vi "Nominal LabVIEW Client API Tree.vi"() -> ()   [LabVIEW 2020]
doc: "This VI is intentionally non-runnable and is designed purely for reference and documentation purposes."
uses:
  Nominal Client.lvclass
  76682c19-609f-4d4f-aff0-eacf46784d00.vi
  2ed37eeb-a64f-4a91-b3eb-4b67bea1485f.vi
  95585ae7-5aba-4d79-b365-cf4aec99f37a.vi
  cba89ab2-b70c-4f15-9195-c2a6f1b0cacd.vi
  95564017-f1d2-4f01-914a-473868c7473e.vi
  f4306f34-5195-4845-a7f4-29a524f2fbc4.vi
  Nominal Client MultiPart Upload/Multipart Upload.lvclass
  timestampMetadata/timestampMetadata.lvclass
  78d8da57-746a-4171-a186-1f17ed8bf924.vi
  ts.epochOfTimeUnit/build.epoch.vi
  ts.epochOfTimeUnit/ts.epochOfTimeUnit.lvclass
  03991706-e7ff-4459-af3d-5364ac0de598.vi
  f1e9a693-645c-4611-911e-4c295cbd5176.vi
  catalog.wait_until_ingest_complete.vi
  ingest_csv.vi
  upload_ingest.csv.vi
  upload_ingest.video.vi
  stream_custom_cluster/stream_custom_cluster.lvclass
  type/type.lvclass
  asset/asset.lvclass
  Run/Run.lvclass
panel:
  in  "Title":string
  in  "data cluster":T1={"Value"=3.14159, "Nanoseconds"=0, "status"=""}
  in  "Description":string
  in  "Dataset Name":string
  # "See Block Diagram"
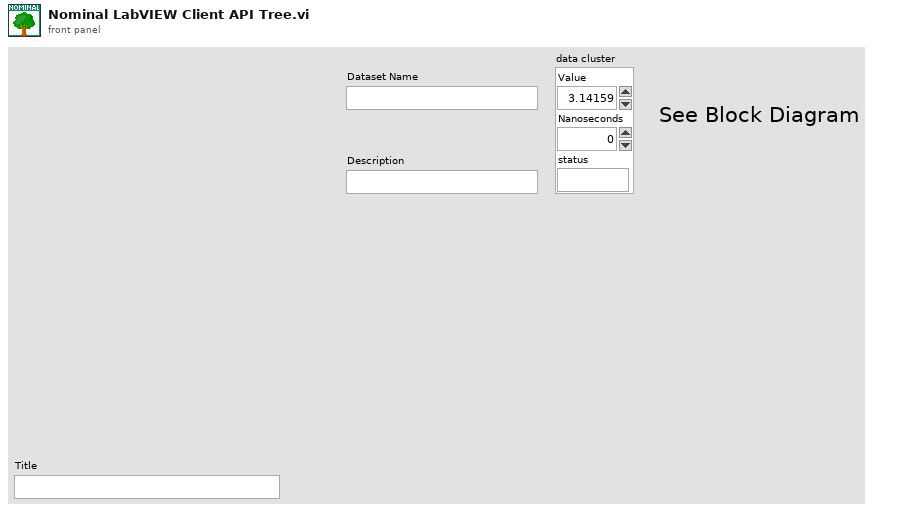
[diagram p1: front panel]
types:
  T1 = cluster{"Value":dbl, "Nanoseconds":i64, "status":string}
  T2 = enum16{"DAYS", "HOURS", "MINUTES", "SECONDS", "MILLISECONDS", "MICROSECONDS", "NANOSECONDS", "PICOSECONDS"}
  T3 = cluster{"Channel":string, "Points":cluster{"UNIX Timestamp":cluster{"Seconds":i64, "Nanoseconds":i64}, "Value":dbl}[]}
  T4 = cluster{"Channel":string, "Points":cluster{"UNIX Timestamp":cluster{"Seconds":i64, "Nanoseconds":i64}, "Value":dbl}[]}[]
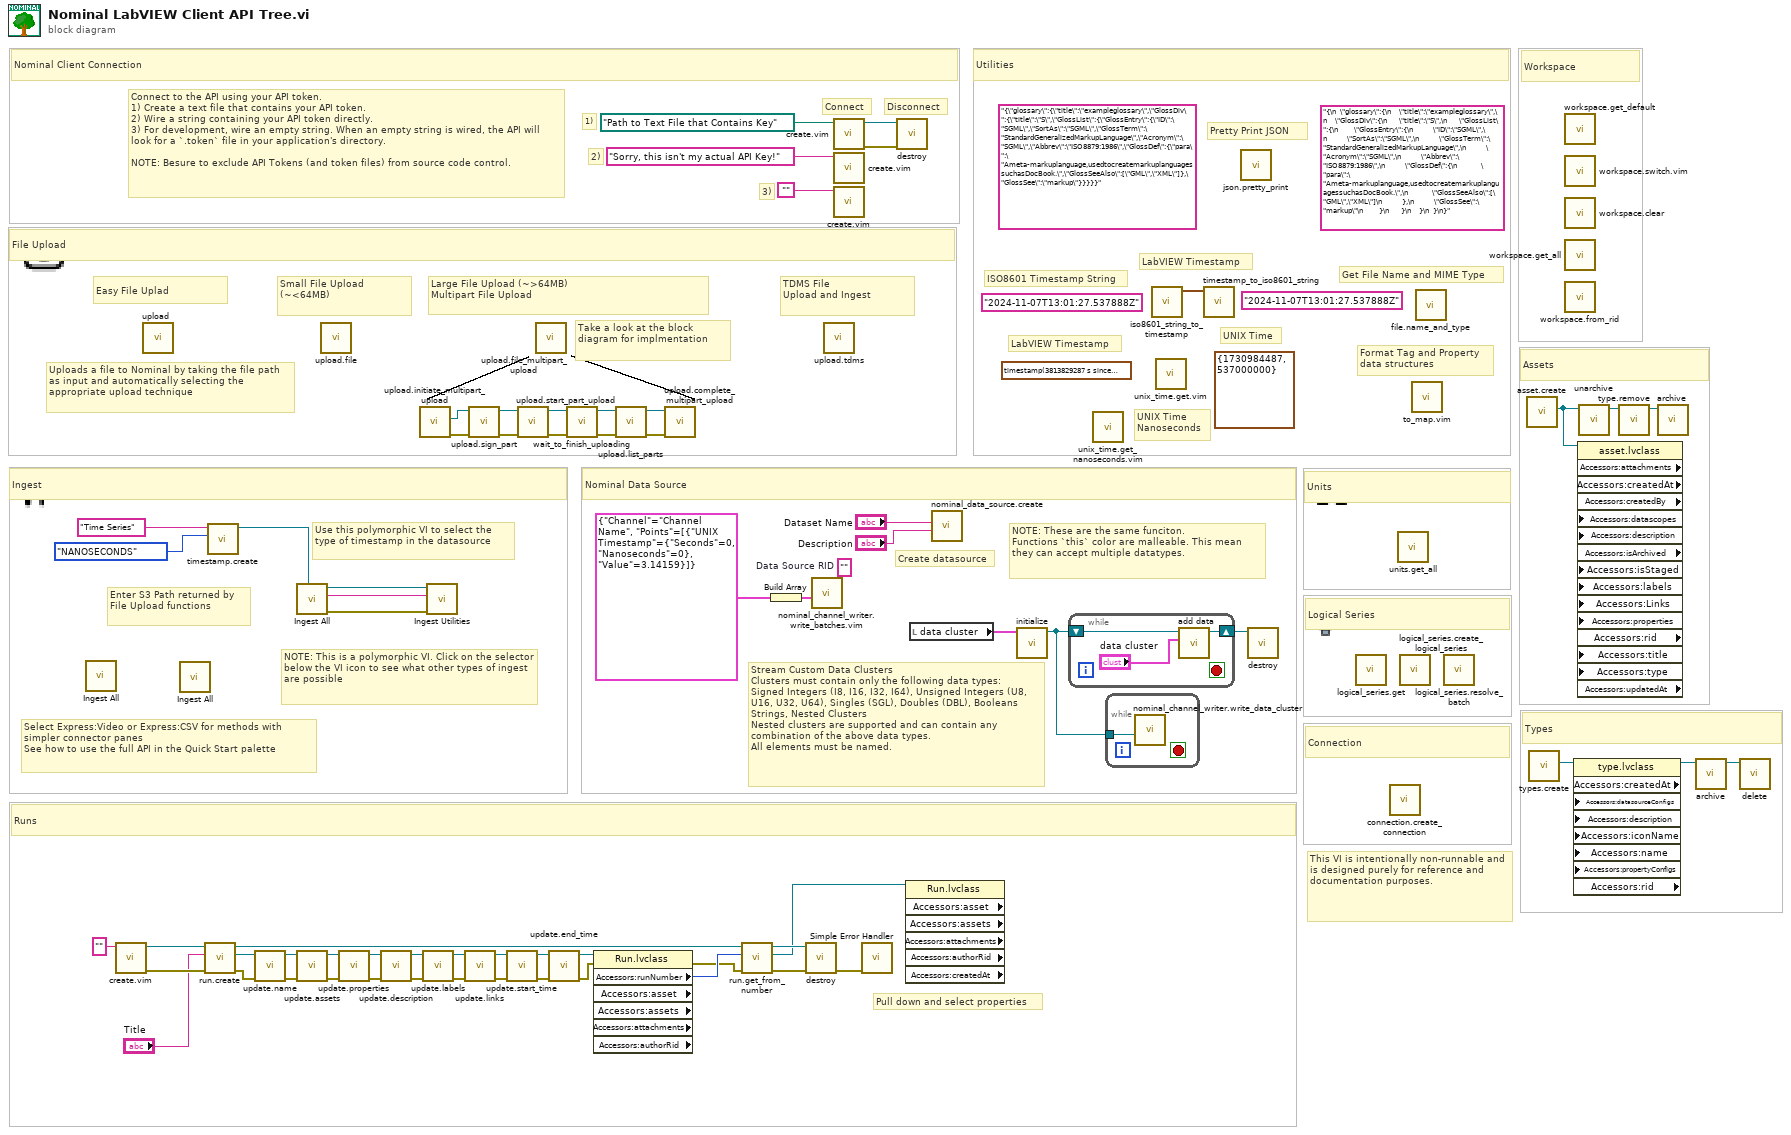
[diagram p0: block diagram]
diagram:
  (unwired) "2024-11-07T13:01:27.537888Z" ("ISO8601 Timestamp String")
  (unwired) ""  # Data Source RID
  (unwired) cluster{"Seconds":i32, "Nanoseconds":i32} {"Seconds"=1730984487, "Nanoseconds"=537000000} ("UNIX Timestamp")
  (unwired) timestamp(3813829287.537 s since 1904-01-01) ("Time Stamp")
  (unwired) "2024-11-07T13:01:27.537888Z" ("ISO8601 Timestamp String")
  (unwired) "{\n  \"glossary\":{\n    \"title\":\"exampleglossary\",\n    \"GlossDiv\":{\n      \"title\":\"S\",\n      \"GlossList\":{\n        \"GlossEntry\":{\n          \"ID\":\"SGML\",\n          \"SortAs\":\"SGML\",\n          \"GlossTerm\":\"StandardGeneralizedMarkupLanguage\",\n          \"Acronym\":\"SGML\",\n          \"Abbrev\":\"ISO8879:1986\",\n          \"GlossDef\":{\n            \"para\":\"Ameta-markuplanguage,usedtocreatemarkuplanguagessuchasDocBook.\",\n            \"GlossSeeAlso\":[\"GML\",\"XML\"]\n          },\n          \"GlossSee\":\"markup\"\n        }\n      }\n    }\n  }\n}"
  (unwired) "{\"glossary\":{\"title\":\"exampleglossary\",\"GlossDiv\":{\"title\":\"S\",\"GlossList\":{\"GlossEntry\":{\"ID\":\"SGML\",\"SortAs\":\"SGML\",\"GlossTerm\":\"StandardGeneralizedMarkupLanguage\",\"Acronym\":\"SGML\",\"Abbrev\":\"ISO8879:1986\",\"GlossDef\":{\"para\":\"Ameta-markuplanguage,usedtocreatemarkuplanguagessuchasDocBook.\",\"GlossSeeAlso\":[\"GML\",\"XML\"]},\"GlossSee\":\"markup\"}}}}}"
  # "Assets"
  # "Types"
  # "Stream Custom Data Clusters\nClusters must contain only the following data types:\nSigned Integers (I8, I16, I32, I64), Unsigned Integers (U8, U16, U32, U64), Singles (SGL), Doubles (DBL), Booleans\nStrings, Nested Clusters\nNested clusters are supported and can contain any combination of the above data types.\nAll elements must be named."
  # "Select Express:Video or Express:CSV for methods with simpler connector panes\nSee how to use the full API in the Quick Start palette"
  # "Workspace"
  # "Connection"
  # "Runs"
  # "Pull down and select properties"
  # "TDMS File\nUpload and Ingest"
  # "This VI is intentionally non-runnable and is designed purely for reference and documentation purposes."
  # "UNIX Time\nNanoseconds"
  # "Format Tag and Property data structures"
  # "Use this polymorphic VI to select the type of timestamp in the datasource"
  # "Easy File Uplad"
  # "Uploads a file to Nominal by taking the file path as input and automatically selecting the appropriate upload technique"
  # "Take a look at the block diagram for implmentation"
  # "NOTE: This is a polymorphic VI. Click on the selector below the VI icon to see what other types of ingest are possible"
  # "Get File Name and MIME Type"
  # "Enter S3 Path returned by File Upload functions"
  # "Ingest"
  # "Pretty Print JSON"
  # "Create datasource"
  # "Disconnect"
  # "Connect"
  # "3)"
  # "2)"
  # "1)"
  # "Connect to the API using your API token.\n1) Create a text file that contains your API token.\n2) Wire a string containing your API token directly.\n3) For development, wire an empty string. When an empty string is wired, the API will look for a `.token` file in your application's directory.\n\nNOTE: Besure to exclude API Tokens (and token files) from source code control."
  # "Nominal Data Source"
  # "NOTE: These are the same funciton.\nFunctions `this` color are malleable. This mean they can accept multiple datatypes."
  # "Large File Upload (~>64MB)\nMultipart File Upload"
  # "Small File Upload\n(~<64MB)"
  # "File Upload"
  # "Nominal Client Connection"
  # "Units"
  # "Logical Series"
  # "Utilities"
  # "UNIX Time"
  # "LabVIEW Timestamp"
  # "LabVIEW Timestamp"
  # "ISO8601 Timestamp String"
  n1 = call-poly "Ingest All.vi"() -> ()  [unwired: 9 in, 3 out]
  n2 = call "create.vim"("API Token (string or path)"="") -> ("error out"=w39:errorcluster, "Nominal Client"=w40:refnum<class "Nominal Client.lvclass">)  [unwired: 8 in, 1 out]
  n3 = call "upload.vi"() -> ()  [unwired: 9 in, 3 out]
  n4 = call-poly "Ingest All.vi"() -> ()  [unwired: 9 in, 3 out]
  n5 = call "run.create.vi"("error in"=w39, "Title"="Title", "Nominal Client in"=w40) -> ("error out"=w1:errorcluster, "Run"=w20:refnum<class "Run.lvclass">, "Nominal Client out"=w2:refnum<class "Nominal Client.lvclass">)  [unwired: 6 in]
  n6 = call-poly "timestamp.create.vi"("Time Unit"=T2."NANOSECONDS", "Time Series Name"="Time Series") -> ("Timestamp Metadata"=w31:refnum<class "timestampMetadata.lvclass">)  [unwired: 9 in]
  n7 = call "update.name.vi"("error in (no error)"=w1, "Run in"=w20) -> ("error out"=w18:errorcluster, "Run out"=w19:refnum<class "Run.lvclass">)  [unwired: 8 in]
  n8 = call-poly "Ingest All.vi"("timestampMetadata"=w31) -> ("error out"=w32:errorcluster, "datasetRid"=w33:string, "Nominal Client out"=w34:refnum<class "Nominal Client.lvclass">)  [unwired: 7 in, 1 out]
  n9 = call "update.assets.vi"("error in (no error)"=w18, "Run in"=w19) -> ("error out"=w16:errorcluster, "Run out"=w17:refnum<class "Run.lvclass">)  [unwired: 8 in]
  n10 = call "upload.file.vi"() -> ()  [unwired: 9 in, 3 out]
  n11 = call "update.properties.vi"("error in (no error)"=w16, "Run in"=w17) -> ("error out"=w14:errorcluster, "Run out"=w15:refnum<class "Run.lvclass">)  [unwired: 8 in]
  n12 = call "update.description.vi"("error in (no error)"=w14, "Run in"=w15) -> ("error out"=w12:errorcluster, "Run out"=w13:refnum<class "Run.lvclass">)  [unwired: 8 in]
  n13 = call "upload.initiate_multipart_upload.vi"() -> ("error out"=w55:errorcluster, "Multipart Upload"=w46:refnum<class "Multipart Upload.lvclass">)  [unwired: 9 in, 1 out]
  n14 = call "update.labels.vi"("error in (no error)"=w12, "Run in"=w13) -> ("error out"=w10:errorcluster, "Run out"=w11:refnum<class "Run.lvclass">)  [unwired: 8 in]
  n15 = call-poly "Ingest Utilities.vi"("error in"=w32, "datasetRid"=w33, "Nominal Client"=w34) -> ()  [unwired: 7 in, 2 out]
  n16 = call "update.links.vi"("error in (no error)"=w10, "Run in"=w11) -> ("error out"=w8:errorcluster, "Run out"=w9:refnum<class "Run.lvclass">)  [unwired: 8 in]
  n17 = call "upload.sign_part.vi"("error in"=w55, "Multipart Upload in"=w46) -> ("error out"=w53:errorcluster, "Multipart Upload out"=w54:refnum<class "Multipart Upload.lvclass">)  [unwired: 8 in]
  n18 = call "update.start_time.vi"("error in (no error)"=w8, "Run in"=w9) -> ("error out"=w6:errorcluster, "Run out"=w7:refnum<class "Run.lvclass">)  [unwired: 8 in]
  n19 = call "upload.start_part_upload.vi"("error in"=w53, "Multipart Upload"=w54) -> ("error out"=w51:errorcluster, "Multipart Upload out"=w52:refnum<class "Multipart Upload.lvclass">)  [unwired: 8 in]
  n20 = call "upload.file_multipart_upload.vi"() -> ()  [unwired: 9 in, 3 out]
  n21 = call "update.end_time.vi"("error in (no error)"=w6, "Run in"=w7) -> ("error out"=w3:errorcluster, "Run out"=w5:refnum<class "Run.lvclass">)  [unwired: 8 in]
  n22 = call "wait_to_finish_uploading.vi"("error in"=w51, "Multipart Upload in"=w52) -> ("error out"=w49:errorcluster, "Multipart Upload out"=w50:refnum<class "Multipart Upload.lvclass">)  [unwired: 8 in]
  n23 = property class="Run.lvclass" props=["Accessors:runNumber", "Accessors:asset", "Accessors:assets", "Accessors:attachments", "Accessors:authorRid"](reference=w5, error in=w3) -> (error out=w4:errorcluster, "Accessors:runNumber"=w36:i32)  [unwired: 5 out]
  n24 = call "upload.list_parts.vi"("error in"=w49, "Multipart Upload"=w50) -> ("error out"=w47:errorcluster, "Multipart Upload out"=w48:refnum<class "Multipart Upload.lvclass">)  [unwired: 8 in]
  n25 = call "upload.complete_multipart_upload.vi"("error in"=w47, "Multipart Upload in"=w48) -> ()  [unwired: 8 in, 2 out]
  n26 = call "run.get_from_number.vi"("error in"=w4, "Run Number"=w36, "Nominal Client in"=w2) -> ("error out"=w37:errorcluster, "Run"=w35:refnum<class "Run.lvclass">, "Nominal Client out"=w38:refnum<class "Nominal Client.lvclass">)  [unwired: 6 in]
  n27 = Build Array(T3 {"Channel"="Channel Name", "Points"=[{"UNIX Timestamp"={"Seconds"=0, "Nanoseconds"=0}, "Value"=3.14159}]}) -> (w61:T4)
  n28 = call "destroy.vi"("error in"=w37, "Nominal Client"=w38) -> ("error out"=w41:errorcluster)  [unwired: 9 in]
  n29 = call "nominal_channel_writer.write_batches.vim"("batches"=w61) -> ()  [unwired: 8 in, 3 out]
  n30 = call "upload.tdms.vi"() -> ()  [unwired: 10 in, 2 out]
  n31 = call "create.vim"("API Token (string or path)"=path "Path to Text File that Contains Key") -> ("error out"=w63:errorcluster, "Nominal Client"=w64:refnum<class "Nominal Client.lvclass">)  [unwired: 8 in, 1 out]
  n32 = call "create.vim"("API Token (string or path)"="Sorry, this isn't my actual API Key!") -> ()  [unwired: 8 in, 3 out]
  n33 = call "create.vim"("API Token (string or path)"="") -> ()  [unwired: 8 in, 3 out]
  n34 = call <vilib>:"Simple Error Handler.vi"("error in (no error)"=w41) -> ()  [unwired: 4 in, 5 out]
  n35 = call "destroy.vi"("error in"=w63, "Nominal Client"=w64) -> ()  [unwired: 9 in, 1 out]
  n36 = property class="Run.lvclass" props=["Accessors:asset", "Accessors:assets", "Accessors:attachments", "Accessors:authorRid", "Accessors:createdAt"](reference=w35) -> ()  [unwired: 1 in, 7 out]
  n37 = local read "data cluster"() -> (w28:T1)
  n38 = call "nominal_data_source.create.vi"("Description"="Description", "Name"="Dataset Name") -> ()  [unwired: 6 in, 4 out]
  n39 = call "initialize.vi"("Data Cluster"=w28) -> ("stream custom cluster"=w29:refnum<class "stream_custom_cluster.lvclass">)  [unwired: 9 in, 1 out]
  n40 = while {
    shift-right: [w66] -> w30
    shift-left: w29 -> [w67]
    stop <- _ stop-if-true
    n41 = call "add data.vi"("Data Cluster"="data cluster", "stream custom cluster in"=w67) -> ("stream custom cluster out"=w66:refnum<class "stream_custom_cluster.lvclass">)  [unwired: 8 in, 1 out]
  }
  n42 = call "unix_time.get_nanoseconds.vim"() -> ()  [unwired: 11 in, 1 out]
  n43 = while {
    tunnel: w29 -> [w68]
    stop <- _ stop-if-true
    n44 = call "nominal_channel_writer.write_data_cluster.vi"("Custom Cluster Streamer"=w68) -> ()  [unwired: 8 in, 3 out]
  }
  n45 = call "iso8601_string_to_timestamp.vi"() -> ("Time Stamp"=w43:timestamp)  [unwired: 10 in, 1 out]
  n46 = call "unix_time.get.vim"() -> ()  [unwired: 11 in, 1 out]
  n47 = call "timestamp_to_iso8601_string.vi"("Time Stamp (now)"=w43) -> ()  [unwired: 10 in, 1 out]
  n48 = call "json.pretty_print.vi"() -> ()  [unwired: 10 in, 2 out]
  n49 = call "destroy.vi"("stream custom cluster"=w30) -> ()  [unwired: 10 in, 1 out]
  n50 = call "logical_series.get.vi"() -> ()  [unwired: 9 in, 3 out]
  n51 = call "connection.create_connection.vi"() -> ()  [unwired: 8 in, 4 out]
  n52 = call "units.get_all.vi"() -> ()  [unwired: 9 in, 3 out]
  n53 = call "logical_series.create_logical_series.vi"() -> ()  [unwired: 9 in, 3 out]
  n54 = call "to_map.vim"() -> ()  [unwired: 11 in, 1 out]
  n55 = call "file.name_and_type.vi"() -> ()  [unwired: 9 in, 3 out]
  n56 = call "logical_series.resolve_batch.vi"() -> ()  [unwired: 9 in, 3 out]
  n57 = call "asset.create.vi"() -> ("asset"=w22:refnum<class "asset.lvclass">)  [unwired: 9 in, 2 out]
  n58 = call "types.create.vi"() -> ("type"=w25:refnum<class "type.lvclass">)  [unwired: 9 in, 2 out]
  n59 = call "workspace.get_default.vi"() -> ()  [unwired: 9 in, 3 out]
  n60 = call "workspace.switch.vim"() -> ()  [unwired: 10 in, 2 out]
  n61 = call "workspace.clear.vi"() -> ()  [unwired: 10 in, 2 out]
  n62 = call "workspace.get_all.vi"() -> ()  [unwired: 9 in, 3 out]
  n63 = call "workspace.from_rid.vi"() -> ()  [unwired: 9 in, 3 out]
  n64 = property class="type.lvclass" props=["Accessors:createdAt", "Accessors:datasourceConfigs", "Accessors:description", "Accessors:iconName", "Accessors:name", "Accessors:propertyConfigs", "Accessors:rid"](reference=w25) -> (reference out=w26:refnum<class "type.lvclass">)  [unwired: 6 in, 3 out]
  n65 = property class="asset.lvclass" props=["Accessors:attachments", "Accessors:createdAt", "Accessors:createdBy", "Accessors:datascopes", "Accessors:description", "Accessors:isArchived", "Accessors:isStaged", "Accessors:labels", "Accessors:Links", "Accessors:properties", "Accessors:rid", "Accessors:title", "Accessors:type", "Accessors:updatedAt"](reference=w22) -> ()  [unwired: 9 in, 8 out]
  n66 = call "unarchive.vi"("asset in"=w22) -> ("asset out"=w23:refnum<class "asset.lvclass">)  [unwired: 9 in, 1 out]
  n67 = call "type.remove.vi"("asset in"=w23) -> ("asset out"=w24:refnum<class "asset.lvclass">)  [unwired: 9 in, 1 out]
  n68 = call "archive.vi"("asset in"=w24) -> ()  [unwired: 9 in, 2 out]
  n69 = call "archive.vi"("type in"=w26) -> ("type out"=w27:refnum<class "type.lvclass">)  [unwired: 9 in, 1 out]
  n70 = call "delete.vi"("type in"=w27) -> ()  [unwired: 9 in, 2 out]
